vi "Go to Node by Path.vi"(8 "error in":errorcluster caption="错误输入（无错误）", 10 "NodePath":string, 11 "PanelLinkNode 输入":refnum<class "PanelLinkNode.lvclass"> caption="DNL_LabVIEW Object in") -> (0 "error out":errorcluster caption="错误输出", 1 "IsRoot?":bool, 2 "Node*":refnum<data-value>, 3 "PanelLinkNode 输出":refnum<class "PanelLinkNode.lvclass"> caption="DNL_LabVIEW Object out")   [LabVIEW 2016, in "PanelLinkNode.lvclass"]
uses:
  PanelLinkNode.lvclass
  PanelObject/PanelObject.lvclass
  PanelLinkNode.lvclass/PanelLinkNode.ctl
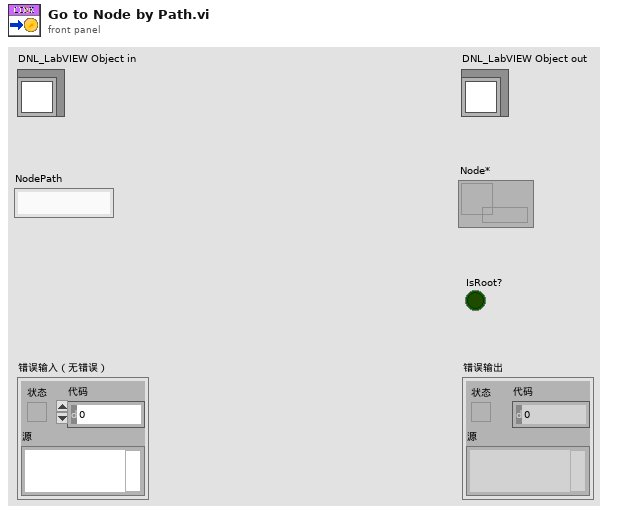
[diagram p1: front panel]
types:
  T1 = cluster{"NodePath/Number":string, "Node*":refnum<data-value>}
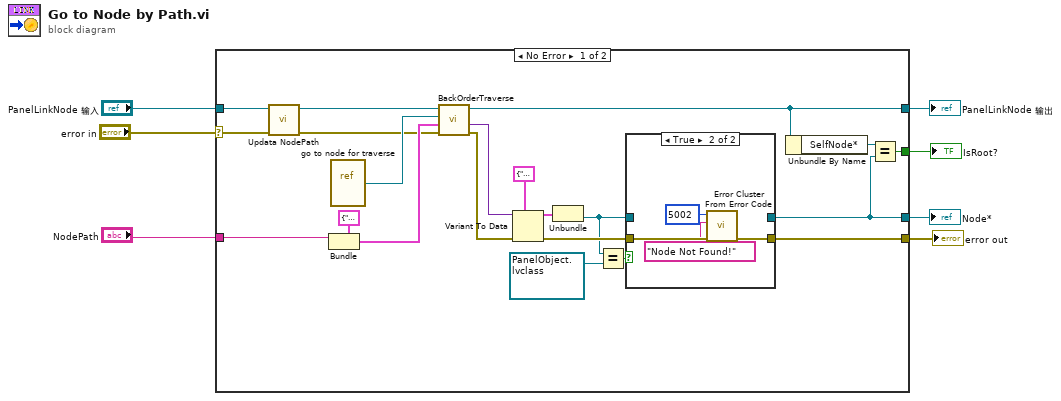
[diagram p0: block diagram]
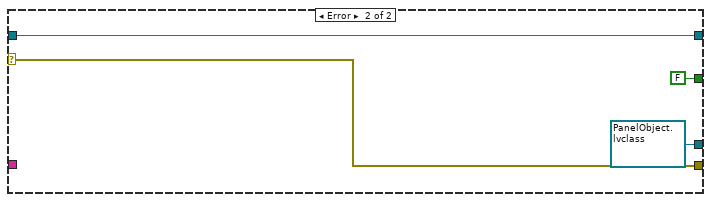
[diagram p3: hidden frame]
diagram:
  n1 = case shown="No Error" "error in" {
    selector: "error in" -> [w8 w38]
    tunnel: [w25 w38] -> w6
    tunnel: [w15 w37] -> w4
    tunnel: "PanelLinkNode 输入" -> [w11 w37]
    tunnel: [w13 refnum<data-value> refnum ("Node*")] -> w1
    tunnel: "NodePath" -> [w22 _]
    tunnel: [w12 FALSE] -> w2
    frame No Error {
      n2 = call-dynamic "Updata NodePath.vi"("error in"=w8, "PanelLinkNode 输入"=w11) -> ("error out"=w9:errorcluster, "PanelLinkNode 输出"=w10:refnum<class "PanelLinkNode.lvclass">)  [unwired: 8 in]
      n3 = Bundle(cluster=T1 {"NodePath/Number"="", "Node*"=refnum} ("Data out"), "NodePath/Number"=w22) -> (w21:T1)  [unwired: 1 in]
      n4 = vi-ref "go to node for traverse.vi"() -> (w16:refnum<vi>)
      n5 = call-dynamic "BackOrderTraverse.vi"("error in"=w9, "Data in"=w21, "vi reference"=w16, "PanelLinkNode 输入"=w10) -> ("error out"=w27:errorcluster, "Data out"=w28:variant, "PanelLinkNode 输出"=w15:refnum<class "PanelLinkNode.lvclass">)  [unwired: 3 in, 2 out]
      n6 = Variant To Data(error in=w27, type=T1 {"NodePath/Number"="", "Node*"=refnum} ("Data out"), Variant=w28) -> (data=w20:T1, error out=w26:errorcluster)
      n7 = Unbundle(w20) -> ("Node*"=w19:refnum<data-value>)  [unwired: 1 out]
      n8 = Equal?(x=w19, y=refnum<data-value> refnum) -> (x = y?=w17:bool)
      n9 = case shown="True" w17 {
        tunnel: [w30 _] -> w13
        tunnel: w26 -> [w29 w33]
        tunnel: [w29 w34] -> w25
        tunnel: w19 -> [w30 _]
        frame False {
        }
        frame True {
          n10 = call <vilib>:"Error Cluster From Error Code.vi"("error in (no error)"=w33, "error message (\"\")"="Node Not Found!" ("error message (\"\")"), "error code (0)"=5002) -> ("error out"=w34:errorcluster)  [unwired: 6 in]
        }
      }
      n11 = Unbundle By Name(w15) -> ("SelfNode*"=w14:refnum<data-value>)
      n12 = Equal?(x=w14, y=w13) -> (x = y?=w12:bool)
    }
    frame Error {
    }
  }
  "error out" <- w6
  "PanelLinkNode 输出" <- w4
  "IsRoot?" <- w2
  "Node*" <- w1
